vi "And Operation (8).vi"(4 "Y":bool[](array[boolean])=[FALSE, FALSE, FALSE, FALSE, FALSE, FALSE, FALSE, FALSE], 5 "X":bool[](array[boolean])=[FALSE, FALSE, FALSE, FALSE, FALSE, FALSE, FALSE, FALSE]) -> (0 "X.and.Y?":bool[](array[boolean]))   [LabVIEW 2011]
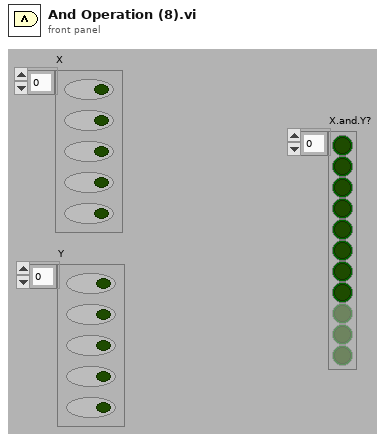
[diagram p1: front panel]
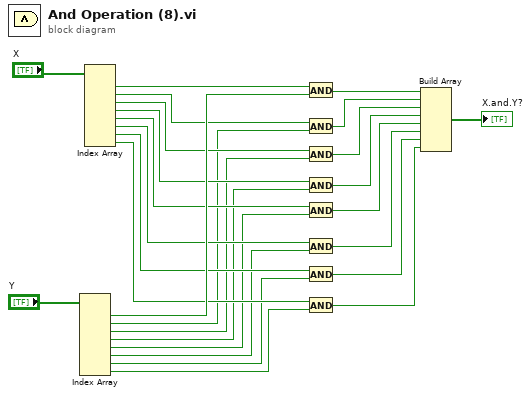
[diagram p0: block diagram]
diagram:
  n1 = Index Array(array="Y") -> (element #1=w24:bool, element #2=w16:bool, element #3=w15:bool, element #4=w14:bool, element #5=w13:bool, element #6=w12:bool, element #7=w11:bool, element #8=w10:bool)  [unwired: 8 in]
  n2 = Index Array(array="X") -> (element #1=w25:bool, element #2=w23:bool, element #3=w22:bool, element #4=w21:bool, element #5=w20:bool, element #6=w19:bool, element #7=w18:bool, element #8=w17:bool)  [unwired: 8 in]
  n3 = And(x=w25, y=w24) -> (x .and. y?=w9:bool)
  n4 = And(x=w23, y=w16) -> (x .and. y?=w8:bool)
  n5 = And(x=w22, y=w15) -> (x .and. y?=w7:bool)
  n6 = And(x=w21, y=w14) -> (x .and. y?=w6:bool)
  n7 = And(x=w20, y=w13) -> (x .and. y?=w5:bool)
  n8 = And(x=w19, y=w12) -> (x .and. y?=w4:bool)
  n9 = And(x=w18, y=w11) -> (x .and. y?=w3:bool)
  n10 = And(x=w17, y=w10) -> (x .and. y?=w2:bool)
  n11 = Build Array(w9, w8, w7, w6, w5, w4, w3, w2) -> (→"X.and.Y?":bool[])
